vi "加标回收启动 (子VI).vi"(11 "启动参数":T1(ring)=enum."CODCr") -> (0 "error out":T2={"status"=FALSE, "代码"=4, "source"=""} caption="错误输出" {"代码" items=["执行成功"=1, "执行失败，但不知道原因"=2, "命令请求条件错误"=3, "通讯超时"=4, "系统繁忙不能执行"=5, "系统故障"=6, "没有数据"=100]})   [LabVIEW 2016]
uses:
  PLC/PLC.lvlib
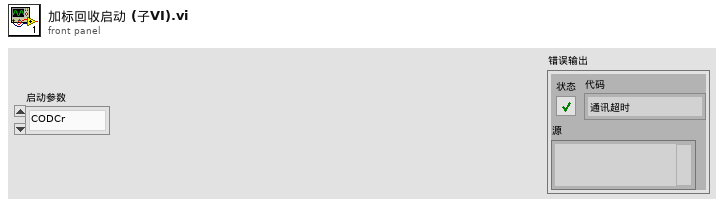
[diagram p1: front panel]
types:
  T1 = enum16{"未选择", "CODMn", "氨氮", "总磷", "总氮", "CODCr"}
  T2 = cluster{"status":bool, "代码":u16, "source":string}
  T3 = enum16{"空闲", "水样测试", "标样核查", "零点核查", "跨度核查", "空白测试", "平行样测试", "质控样", "空白校准", "标样校准", "加标回收"}
  T4 = enum16{"空闲", "水样测试", "标样核查", "零点核查", "跨度核查", "空白测试", "平行样测试", "加标回收", "空白校准", "标样校准", "初始化（清洗）"}
  T5 = cluster{"是否启用仪器":bool, "CODMn":cluster{"启动测量模式":cluster{"测量模式":enum16{"水样测量", "标样核查", "加标回收", "平行样", "校零", "校标"}}, "确定按钮":bool}, "启动模块":cluster{"氨氮":bool, "总磷":bool, "总氮":bool, "COD":bool}, "常规启动":bool, "直接启动":bool}
  T6 = cluster{"R0":i16, "R1":i16, "R2":i16, "R3":i16, "R4":i16, "R5":i16, "R6":i16, "R7":i16, "R8":i16, "R9":i16, "R10":i16, "R11":i16, "R12":i16, "R13":i16, "R14":i16, "R15":i16, "R16":i16, "R17":i16, "R18":i16, "R19":i16, "R20":i16, "R21":i16, "R22":i16, "R23":i16, "R24":i16, "R25":i16, "R26":i16, "R27":i16, "R28":i16, "R29":i16, "R30":i16, "R31":i16, "R32":i16, "R33":i16, "R34":i16}
  T7 = enum32{"Bad", "Idle", "Run top level", "Running"}
  T8 = cluster{"系统时间":timestamp, "工作状态":enum16{"空闲", "水样测试", "标样核查", "零点核查", "跨度核查", "空白测试", "平行样测试", "加标回收", "空白校准", "标样校准", "初始化（清洗）"}, "测量模式":enum16{"待机", "连续模式", "周期模式", "定点模式", "受控模式", "手动模式"}, "告警代码":u16, "故障代码":u16, "日志代码":u16, "软件版本":u16, "F0":sgl, "F1":sgl, "F2":sgl, "F3":sgl, "T":sgl, "H":sgl, "id":u16, "flowid":u16, "量程":u16, "总磷控温温度1":sgl, "营养盐控温温度2":sgl, "ADC":sgl}
  T9 = cluster{"系统时间":timestamp, "工作状态":u16, "测量模式":u16, "告警代码":enum16{"无告警", "缺试剂告警", "缺水样告警", "缺蒸馏水告警", "缺标液告警", "仪表漏液告警", "标定异常告警", "超量程告警", "加热异常", "低试剂预警", "超上限告警", "超下限告警", "仪表内部其他异常", "滴定异常告警", "电极异常告警", "量程切换告警", "参数设置告警", "PH电极电位异常", "电导率电极异常", "浊度光度异常", "溶解氧电极异常", "溶解氧光强异常", "温度异常告警", "PH异常告警", "溶解氧异常告警", "电导率异常告警", "浊度异常告警", "叶绿素异常告警", "藻密度异常告警", "蓝绿藻异常告警", "ORP异常告警", "氨氮异常告警", "清洁刷异常告警", "SD卡异常告警", "蓝牙异常告警", "Wifi异常告警", "流程异常告警"}, "故障代码":enum16{"无故障", "电机故障", "温度故障", "通讯故障", "滴定故障"}, "日志代码":u16, "软件版本":u16, "F0":sgl, "F1":sgl, "F2":sgl, "F3":sgl, "T":sgl, "H":sgl, "id":u16, "flowid":u16, "量程":u16}
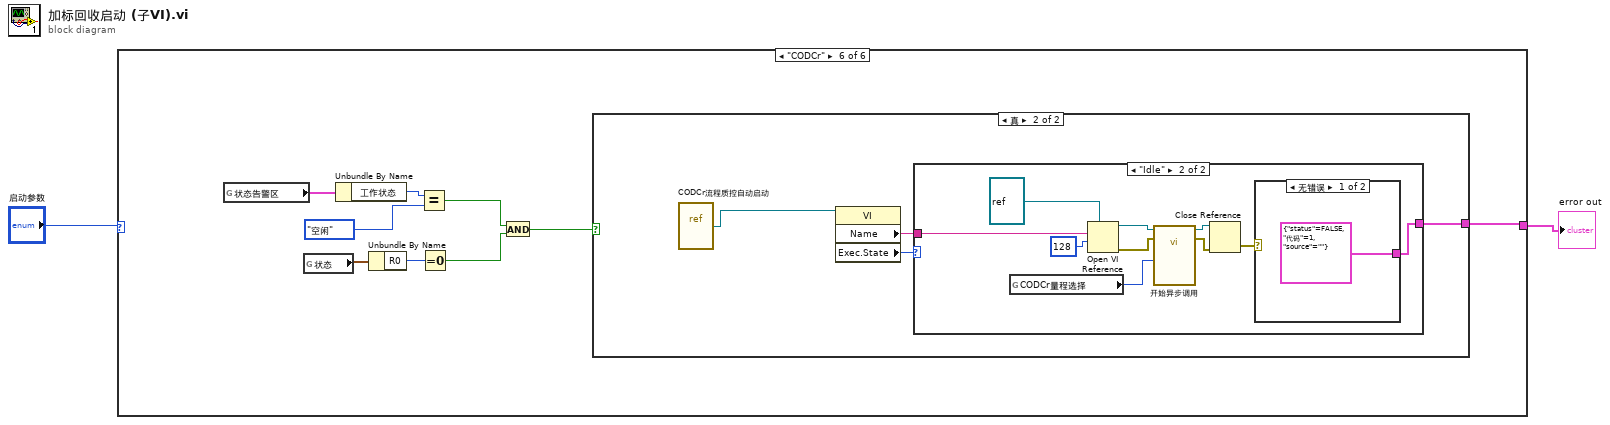
[diagram p0: block diagram]
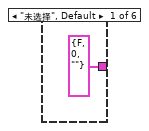
[diagram p2: hidden frame]
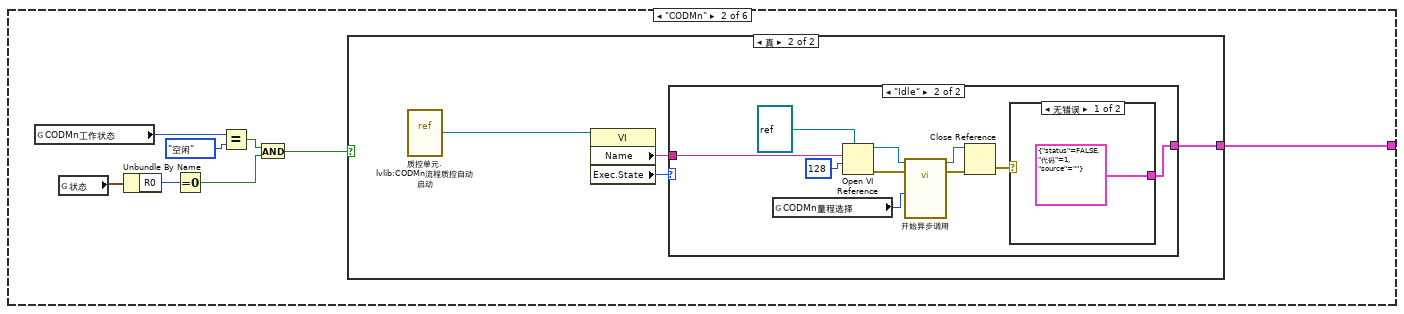
[diagram p3: hidden frame]
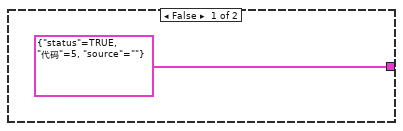
[diagram p4: hidden frame]
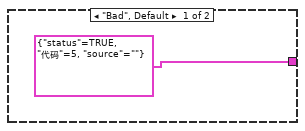
[diagram p5: hidden frame]
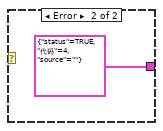
[diagram p6: hidden frame]
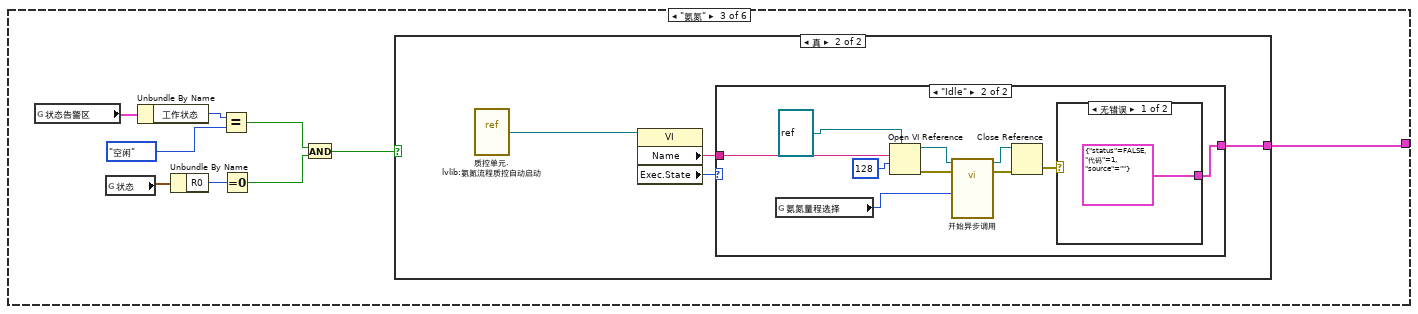
[diagram p7: hidden frame]
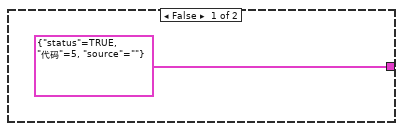
[diagram p8: hidden frame]
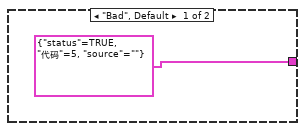
[diagram p9: hidden frame]
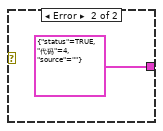
[diagram p10: hidden frame]
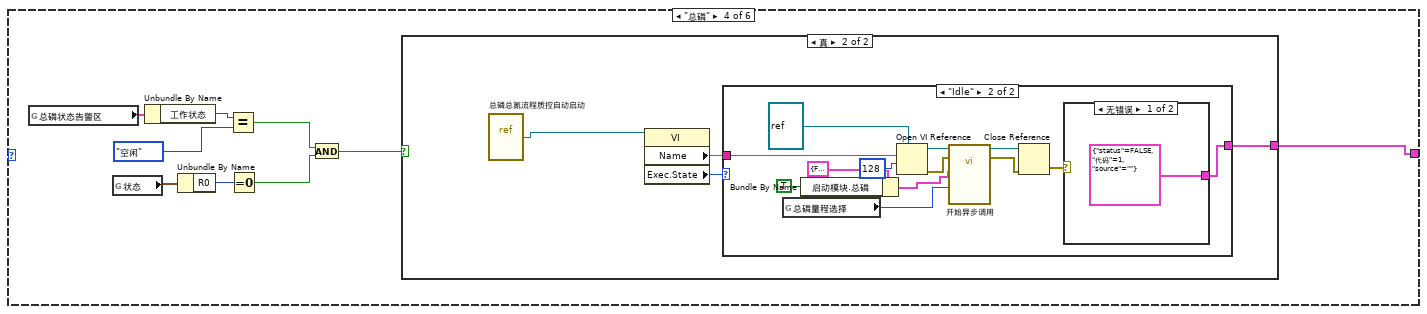
[diagram p11: hidden frame]
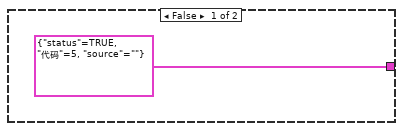
[diagram p12: hidden frame]
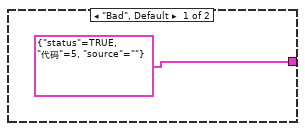
[diagram p13: hidden frame]
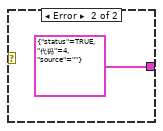
[diagram p14: hidden frame]
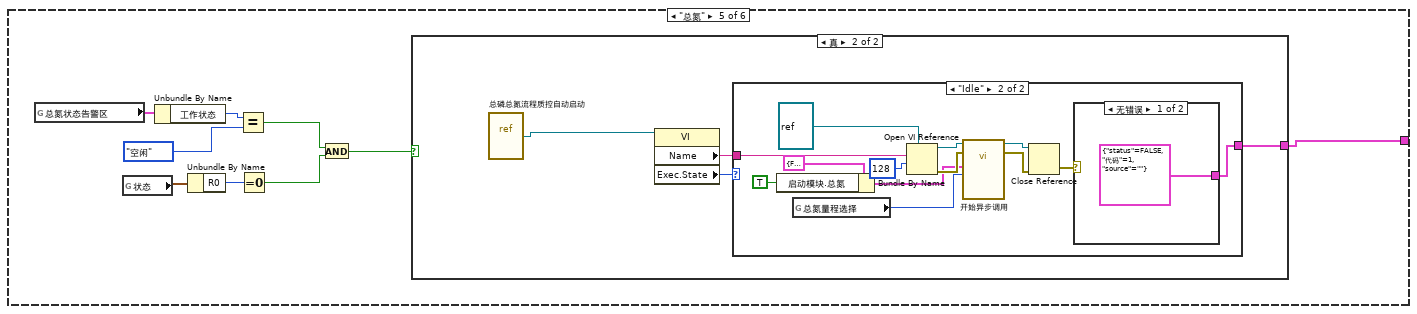
[diagram p15: hidden frame]
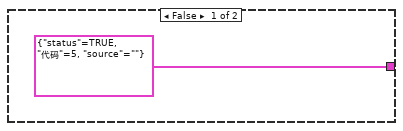
[diagram p16: hidden frame]
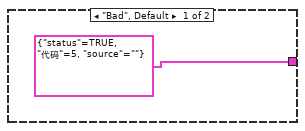
[diagram p17: hidden frame]
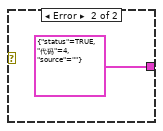
[diagram p18: hidden frame]
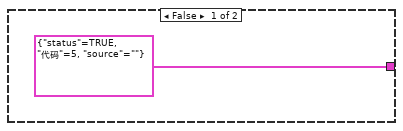
[diagram p19: hidden frame]
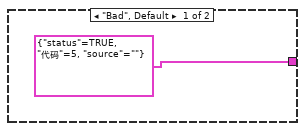
[diagram p20: hidden frame]
diagram:
  n1 = case shown="\"CODCr\"" "启动参数" {
    tunnel: [T2 {"status"=FALSE, "代码"=0, "source"=""} ("error out") w4 w34 w58 w87 w118] -> w1
    frame "未选择", Default {
    }
    frame "CODMn" {
      n2 = global read "COD测量模式全局.vi" "CODMn工作状态"() -> (w11:T3)
      n3 = global read "采配水全局变量.vi" "状态"() -> (w8:T6)
      n4 = Unbundle By Name(w8) -> ("R0"=w7:i16)
      n5 = Equal To 0?(x=w7) -> (x = 0?=w6:bool)
      n6 = Equal?(x=w11, y=T3."空闲") -> (x = y?=w9:bool)
      n7 = And(x=w9, y=w6) -> (x .and. y?=w5:bool)
      n8 = case shown="真" w5 {
        tunnel: [T2 {"status"=TRUE, "代码"=5, "source"=""} ("error out") w13] -> w4
        frame False {
        }
        frame True {
          n9 = vi-ref "质控单元.lvlib:CODMn流程质控自动启动.vi"() -> (w14:refnum<vi>)
          n10 = property class="VI"(reference=w14) -> ("Name"=w16:string, "Exec.State"=w15:T7)  [unwired: 1 in, 2 out]
          n11 = case shown="\"Idle\"" w15 {
            tunnel: w16 -> [_ w24]
            tunnel: [T2 {"status"=TRUE, "代码"=5, "source"=""} ("error out") w20] -> w13
            frame "Bad", Default {
            }
            frame "Idle" {
              n12 = global read "断电保存全局.vi" "CODMn量程选择"() -> (w18:enum32{"H", "L", "AUTO"})
              n13 = Open VI Reference(type specifier VI Refnum (for type only)=refnum<vi> refnum ("类型说明符VI引用句柄（仅用于类型）"), vi path=w24, options=128 ("选项")) -> (vi reference=w19:refnum<vi>, error out=w23:errorcluster)  [unwired: 3 in]
              n14 = call-by-ref "开始异步调用"(reference=w19, error in=w23, "CODMn量程切换"=w18) -> (reference out=w27:refnum<vi>, error out=w22:errorcluster)  [unwired: 10 in]
              n15 = Close Reference(reference=w27, error in (no error)=w22) -> (error out=w21:errorcluster)
              n16 = case shown="无错误" w21 {
                tunnel: [T2 {"status"=FALSE, "代码"=1, "source"=""} ("error out") T2 {"status"=TRUE, "代码"=4, "source"=""} ("error out")] -> w20
                frame No Error {
                }
                frame Error {
                }
              }
            }
          }
        }
      }
    }
    frame "氨氮" {
      n17 = global read "VAR氨氮全局变量.vi" "状态告警区"() -> (w33:T8)
      n18 = global read "采配水全局变量.vi" "状态"() -> (w38:T6)
      n19 = Unbundle By Name(w33) -> ("工作状态"=w32:T4)
      n20 = Unbundle By Name(w38) -> ("R0"=w37:i16)
      n21 = Equal?(x=w32, y=T4."空闲") -> (x = y?=w30:bool)
      n22 = Equal To 0?(x=w37) -> (x = 0?=w36:bool)
      n23 = And(x=w30, y=w36) -> (x .and. y?=w35:bool)
      n24 = case shown="真" w35 {
        tunnel: [T2 {"status"=TRUE, "代码"=5, "source"=""} ("error out") w41] -> w34
        frame False {
        }
        frame True {
          n25 = vi-ref "质控单元.lvlib:氨氮流程质控自动启动.vi"() -> (w40:refnum<vi>)
          n26 = property class="VI"(reference=w40) -> ("Name"=w43:string, "Exec.State"=w42:T7)  [unwired: 1 in, 2 out]
          n27 = case shown="\"Idle\"" w42 {
            tunnel: w43 -> [_ w51]
            tunnel: [T2 {"status"=TRUE, "代码"=5, "source"=""} ("error out") w47] -> w41
            frame "Bad", Default {
            }
            frame "Idle" {
              n28 = global read "断电保存全局.vi" "氨氮量程选择"() -> (w45:enum32{"H", "L", "AUTO"})
              n29 = Open VI Reference(type specifier VI Refnum (for type only)=refnum<vi> refnum ("类型说明符VI引用句柄（仅用于类型）"), vi path=w51, options=128 ("选项")) -> (vi reference=w54:refnum<vi>, error out=w50:errorcluster)  [unwired: 3 in]
              n30 = call-by-ref "开始异步调用"(reference=w54, error in=w50, "氨氮量程切换"=w45) -> (reference out=w53:refnum<vi>, error out=w49:errorcluster)  [unwired: 11 in]
              n31 = Close Reference(reference=w53, error in (no error)=w49) -> (error out=w48:errorcluster)
              n32 = case shown="无错误" w48 {
                tunnel: [T2 {"status"=FALSE, "代码"=1, "source"=""} ("error out") T2 {"status"=TRUE, "代码"=4, "source"=""} ("error out")] -> w47
                frame No Error {
                }
                frame Error {
                }
              }
            }
          }
        }
      }
    }
    frame "总磷" {
      n33 = global read "VAR总磷总氮全局变量.vi" "总磷状态告警区"() -> (w57:T8)
      n34 = global read "采配水全局变量.vi" "状态"() -> (w65:T6)
      n35 = Unbundle By Name(w57) -> ("工作状态"=w61:T4)
      n36 = Unbundle By Name(w65) -> ("R0"=w64:i16)
      n37 = Equal?(x=w61, y=T4."空闲") -> (x = y?=w59:bool)
      n38 = Equal To 0?(x=w64) -> (x = 0?=w63:bool)
      n39 = And(x=w59, y=w63) -> (x .and. y?=w62:bool)
      n40 = case shown="真" w62 {
        tunnel: [T2 {"status"=TRUE, "代码"=5, "source"=""} ("error out") w68] -> w58
        frame False {
        }
        frame True {
          n41 = vi-ref "总磷总氮流程质控自动启动.vi"() -> (w67:refnum<vi>)
          n42 = property class="VI"(reference=w67) -> ("Name"=w70:string, "Exec.State"=w69:T7)  [unwired: 1 in, 2 out]
          n43 = case shown="\"Idle\"" w69 {
            tunnel: w70 -> [_ w83]
            tunnel: [T2 {"status"=TRUE, "代码"=5, "source"=""} ("error out") w80] -> w68
            frame "Bad", Default {
            }
            frame "Idle" {
              n44 = global read "断电保存全局.vi" "总磷量程选择"() -> (w75:enum32{"H", "L", "AUTO"})
              n45 = Bundle By Name(cluster=T5 {"是否启用仪器"=FALSE, "CODMn"={"启动测量模式"={"测量模式"=enum."水样测量"}, "确定按钮"=FALSE}, "启动模块"={"氨氮"=FALSE, "总磷"=FALSE, "总氮"=FALSE, "COD"=FALSE}, "常规启动"=FALSE, "直接启动"=FALSE} ("参数"), "启动模块.总磷"=TRUE) -> (w72:T5)
              n46 = Open VI Reference(type specifier VI Refnum (for type only)=refnum<vi> refnum ("类型说明符VI引用句柄（仅用于类型）"), vi path=w83, options=128 ("选项")) -> (vi reference=w78:refnum<vi>, error out=w77:errorcluster)  [unwired: 3 in]
              n47 = call-by-ref "开始异步调用"(reference=w78, error in=w77, "总磷量程切换"=w75, "参数"=w72) -> (reference out=w76:refnum<vi>, error out=w82:errorcluster)  [unwired: 10 in]
              n48 = Close Reference(reference=w76, error in (no error)=w82) -> (error out=w81:errorcluster)
              n49 = case shown="无错误" w81 {
                tunnel: [T2 {"status"=FALSE, "代码"=1, "source"=""} ("error out") T2 {"status"=TRUE, "代码"=4, "source"=""} ("error out")] -> w80
                frame No Error {
                }
                frame Error {
                }
              }
            }
          }
        }
      }
    }
    frame "总氮" {
      n50 = global read "VAR总磷总氮全局变量.vi" "总氮状态告警区"() -> (w88:T8)
      n51 = global read "采配水全局变量.vi" "状态"() -> (w95:T6)
      n52 = Unbundle By Name(w88) -> ("工作状态"=w91:T4)
      n53 = Unbundle By Name(w95) -> ("R0"=w94:i16)
      n54 = Equal?(x=w91, y=T4."空闲") -> (x = y?=w89:bool)
      n55 = Equal To 0?(x=w94) -> (x = 0?=w93:bool)
      n56 = And(x=w89, y=w93) -> (x .and. y?=w92:bool)
      n57 = case shown="真" w92 {
        tunnel: [T2 {"status"=TRUE, "代码"=5, "source"=""} ("error out") w98] -> w87
        frame False {
        }
        frame True {
          n58 = vi-ref "总磷总氮流程质控自动启动.vi"() -> (w97:refnum<vi>)
          n59 = property class="VI"(reference=w97) -> ("Name"=w100:string, "Exec.State"=w99:T7)  [unwired: 1 in, 2 out]
          n60 = case shown="\"Idle\"" w99 {
            tunnel: w100 -> [_ w113]
            tunnel: [T2 {"status"=TRUE, "代码"=5, "source"=""} ("error out") w111] -> w98
            frame "Bad", Default {
            }
            frame "Idle" {
              n61 = Bundle By Name(cluster=T5 {"是否启用仪器"=FALSE, "CODMn"={"启动测量模式"={"测量模式"=enum."水样测量"}, "确定按钮"=FALSE}, "启动模块"={"氨氮"=FALSE, "总磷"=FALSE, "总氮"=FALSE, "COD"=FALSE}, "常规启动"=FALSE, "直接启动"=FALSE} ("参数"), "启动模块.总氮"=TRUE) -> (w102:T5)
              n62 = global read "断电保存全局.vi" "总氮量程选择"() -> (w107:enum32{"H", "L", "AUTO"})
              n63 = Open VI Reference(type specifier VI Refnum (for type only)=refnum<vi> refnum ("类型说明符VI引用句柄（仅用于类型）"), vi path=w113, options=128 ("选项")) -> (vi reference=w109:refnum<vi>, error out=w108:errorcluster)  [unwired: 3 in]
              n64 = call-by-ref "开始异步调用"(reference=w109, error in=w108, "总氮量程切换"=w107, "参数"=w102) -> (reference out=w106:refnum<vi>, error out=w105:errorcluster)  [unwired: 10 in]
              n65 = Close Reference(reference=w106, error in (no error)=w105) -> (error out=w112:errorcluster)
              n66 = case shown="无错误" w112 {
                tunnel: [T2 {"status"=FALSE, "代码"=1, "source"=""} ("error out") T2 {"status"=TRUE, "代码"=4, "source"=""} ("error out")] -> w111
                frame No Error {
                }
                frame Error {
                }
              }
            }
          }
        }
      }
    }
    frame "CODCr" {
      n67 = global read "CODcr全局变量.vi" "状态告警区"() -> (w117:T9)
      n68 = global read "采配水全局变量.vi" "状态"() -> (w125:T6)
      n69 = Unbundle By Name(w117) -> ("工作状态"=w121:u16)
      n70 = Unbundle By Name(w125) -> ("R0"=w124:i16)
      n71 = Equal?(x=w121, y=T4."空闲") -> (x = y?=w119:bool)
      n72 = Equal To 0?(x=w124) -> (x = 0?=w123:bool)
      n73 = And(x=w119, y=w123) -> (x .and. y?=w122:bool)
      n74 = case shown="真" w122 {
        tunnel: [T2 {"status"=TRUE, "代码"=5, "source"=""} ("error out") w128] -> w118
        frame False {
        }
        frame True {
          n75 = vi-ref "CODCr流程质控自动启动.vi"() -> (w127:refnum<vi>)
          n76 = property class="VI"(reference=w127) -> ("Name"=w130:string, "Exec.State"=w129:T7)  [unwired: 1 in, 2 out]
          n77 = case shown="\"Idle\"" w129 {
            tunnel: w130 -> [_ w140]
            tunnel: [T2 {"status"=TRUE, "代码"=5, "source"=""} ("error out") w138] -> w128
            frame "Bad", Default {
            }
            frame "Idle" {
              n78 = global read "断电保存全局.vi" "CODCr量程选择"() -> (w135:enum32{"H", "L", "AUTO"})
              n79 = Open VI Reference(type specifier VI Refnum (for type only)=refnum<vi> refnum ("类型说明符VI引用句柄（仅用于类型）"), vi path=w140, options=128 ("选项")) -> (vi reference=w136:refnum<vi>, error out=w134:errorcluster)  [unwired: 3 in]
              n80 = call-by-ref "开始异步调用"(reference=w136, error in=w134, "CODCr量程切换"=w135) -> (reference out=w133:refnum<vi>, error out=w132:errorcluster)  [unwired: 10 in]
              n81 = Close Reference(reference=w133, error in (no error)=w132) -> (error out=w139:errorcluster)
              n82 = case shown="无错误" w139 {
                tunnel: [T2 {"status"=FALSE, "代码"=1, "source"=""} ("error out") T2 {"status"=TRUE, "代码"=4, "source"=""} ("error out")] -> w138
                frame No Error {
                }
                frame Error {
                }
              }
            }
          }
        }
      }
    }
  }
  "error out" <- w1
